vi "CanCoder_Begin.vi"   [LabVIEW 2023]
uses:
  <vilib>/Rock Robotics/WPI/ThirdParty/Phoenix-LabVIEW/CANCoder/Controls/CTRE_Phoenix_CANcoder_SensorTimeBase.ctl
types:
  T1 = typedef "CTRE_Phoenix_CANcoder_SensorTimeBase.ctl" = enum16{"Per100Ms_Legacy", "PerSecond", "PerMinute"}
  T2 = typedef "CTRE_Phoenix_CANcoder_DeviceRef.ctl" = cluster{"DeviceStatus":errorcluster, "Device Number":u8, "Handle":u64, "UsageFrame":u32, "Library Path":path}
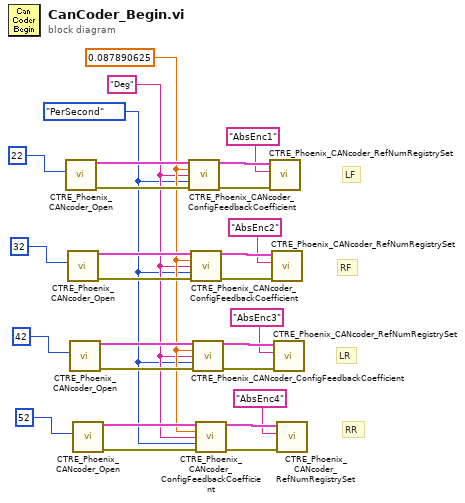
[diagram p0: block diagram]
diagram:
  w1 = CTRE_Phoenix_CANcoder_SensorTimeBase."PerSecond" ("timebase")
  w2 = "Deg" ("unitString")
  w3 = 0.087890625 ("sensorCoefficient")
  # "RR"
  # "LR"
  # "RF"
  # "LF"
  n1 = call <vilib>:"CTRE_Phoenix_CANcoder_Open.vi"("Device Number"=u8 22) -> ("error out"=w22:errorcluster, "CTRE_CANcoder_DeviceRef"=w26:T2)  [unwired: 9 in]
  n2 = call <vilib>:"CTRE_Phoenix_CANcoder_Open.vi"("Device Number"=u8 32) -> ("error out"=w16:errorcluster, "CTRE_CANcoder_DeviceRef"=w20:T2)  [unwired: 9 in]
  n3 = call <vilib>:"CTRE_Phoenix_CANcoder_Open.vi"("Device Number"=u8 42) -> ("error out"=w10:errorcluster, "CTRE_CANcoder_DeviceRef"=w14:T2)  [unwired: 9 in]
  n4 = call <vilib>:"CTRE_Phoenix_CANcoder_Open.vi"("Device Number"=u8 52) -> ("error out"=w4:errorcluster, "CTRE_CANcoder_DeviceRef"=w8:T2)  [unwired: 9 in]
  n5 = call <vilib>:"CTRE_Phoenix_CANcoder_ConfigFeedbackCoefficient.vi"("CTRE_CANcoder_DeviceRef"=w26, "sensorCoefficient"=w3, "unitString"=w2, "timebase"=w1, "error in"=w22) -> ("CTRE_CANcoder_DeviceRef"=w25:T2, "error out"=w24:errorcluster)  [unwired: 9 in]
  n6 = call <vilib>:"CTRE_Phoenix_CANcoder_ConfigFeedbackCoefficient.vi"("CTRE_CANcoder_DeviceRef"=w20, "sensorCoefficient"=w3, "unitString"=w2, "timebase"=w1, "error in"=w16) -> ("CTRE_CANcoder_DeviceRef"=w19:T2, "error out"=w18:errorcluster)  [unwired: 9 in]
  n7 = call <vilib>:"CTRE_Phoenix_CANcoder_ConfigFeedbackCoefficient.vi"("CTRE_CANcoder_DeviceRef"=w14, "sensorCoefficient"=w3, "unitString"=w2, "timebase"=w1, "error in"=w10) -> ("CTRE_CANcoder_DeviceRef"=w13:T2, "error out"=w12:errorcluster)  [unwired: 9 in]
  n8 = call <vilib>:"CTRE_Phoenix_CANcoder_ConfigFeedbackCoefficient.vi"("CTRE_CANcoder_DeviceRef"=w8, "sensorCoefficient"=w3, "unitString"=w2, "timebase"=w1, "error in"=w4) -> ("CTRE_CANcoder_DeviceRef"=w7:T2, "error out"=w6:errorcluster)  [unwired: 9 in]
  n9 = call <vilib>:"CTRE_Phoenix_CANcoder_RefNumRegistrySet.vi"("error in (no error)"=w24, "refnum name"="AbsEnc1", "CTRE_CANcoder_DeviceRef"=w25) -> ()  [unwired: 7 in, 2 out]
  n10 = call <vilib>:"CTRE_Phoenix_CANcoder_RefNumRegistrySet.vi"("error in (no error)"=w18, "refnum name"="AbsEnc2", "CTRE_CANcoder_DeviceRef"=w19) -> ()  [unwired: 7 in, 2 out]
  n11 = call <vilib>:"CTRE_Phoenix_CANcoder_RefNumRegistrySet.vi"("error in (no error)"=w12, "refnum name"="AbsEnc3", "CTRE_CANcoder_DeviceRef"=w13) -> ()  [unwired: 7 in, 2 out]
  n12 = call <vilib>:"CTRE_Phoenix_CANcoder_RefNumRegistrySet.vi"("error in (no error)"=w6, "refnum name"="AbsEnc4", "CTRE_CANcoder_DeviceRef"=w7) -> ()  [unwired: 7 in, 2 out]
